vi "softwareTriggerInstructionFA.vi"(8 "error in (no error)":errorcluster, 10 "ModbusBuffer in":refnum<class "ModbusBuffer.lvclass">, 11 "ILCCommunications in":refnum<class "ILCCommunications.lvclass">) -> (0 "error out":errorcluster, 2 "ModbusBuffer out":refnum<class "ModbusBuffer.lvclass">, 3 "ILCCommunications out":refnum<class "ILCCommunications.lvclass">)   [LabVIEW 2016, in "ILCCommunications.lvclass"]
uses:
  ILCCommunications.lvclass
  Common_RT_Modbus/ModbusBuffer/ModbusBuffer.lvclass
  Common_RT_Modbus/ModbusBuffer/ModbusBuffer.lvclass/ModbusBuffer.ctl
  Common_RT_Modbus/ModbusBuffer/writeSoftwareTrigger.vi
  Common_RT_Modbus/ModbusBuffer/writeHeader.vi
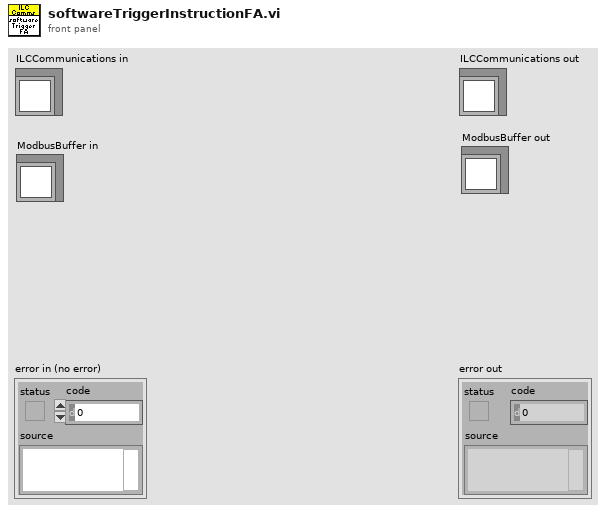
[diagram p1: front panel]
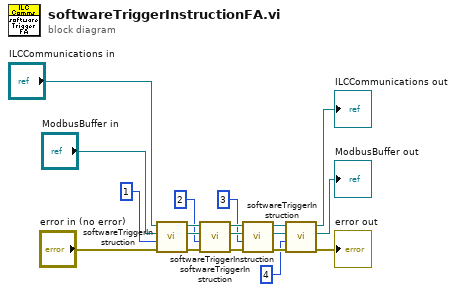
[diagram p0: block diagram]
diagram:
  n1 = call "softwareTriggerInstruction.vi"("error in (no error)"="error in (no error)", "Subnet"=u8 1, "ModbusBuffer in"="ModbusBuffer in", "ILCCommunications in"="ILCCommunications in") -> ("error out"=w16:errorcluster, "ModbusBuffer out"=w15:refnum<class "ModbusBuffer.lvclass">, "ILCCommunications out"=w14:refnum<class "ILCCommunications.lvclass">)  [unwired: 5 in]
  n2 = call "softwareTriggerInstruction.vi"("error in (no error)"=w16, "Subnet"=u8 2, "ModbusBuffer in"=w15, "ILCCommunications in"=w14) -> ("error out"=w13:errorcluster, "ModbusBuffer out"=w12:refnum<class "ModbusBuffer.lvclass">, "ILCCommunications out"=w11:refnum<class "ILCCommunications.lvclass">)  [unwired: 5 in]
  n3 = call "softwareTriggerInstruction.vi"("error in (no error)"=w13, "Subnet"=u8 3, "ModbusBuffer in"=w12, "ILCCommunications in"=w11) -> ("error out"=w10:errorcluster, "ModbusBuffer out"=w9:refnum<class "ModbusBuffer.lvclass">, "ILCCommunications out"=w8:refnum<class "ILCCommunications.lvclass">)  [unwired: 5 in]
  n4 = call "softwareTriggerInstruction.vi"("error in (no error)"=w10, "Subnet"=u8 4, "ModbusBuffer in"=w9, "ILCCommunications in"=w8) -> ("error out"=→"error out":errorcluster, "ModbusBuffer out"=→"ModbusBuffer out":refnum<class "ModbusBuffer.lvclass">, "ILCCommunications out"=→"ILCCommunications out":refnum<class "ILCCommunications.lvclass">)  [unwired: 5 in]
